vi "Compile - Rx Packet Information.vi"(8 "error in (no error)":errorcluster, 11 "Custom Device Ref in":T1 format="%.0x") -> (0 "error out":errorcluster, 1 "Rx Ref Array":T2(array[cluster]) {"VS Refs" format="%.0x"}, 2 "Rx Packet Info Array":T3[](array[typedef]) {"Endianness" items=["big-endian"=0, "little-indian"=2]}, 3 "Custom Device Ref out":T1 format="%.0x")   [LabVIEW 2019, in "UDP-Custom-Device System Explorer.lvlib"]
uses:
  UDP-Custom-Device System Explorer.lvlib
  Shared/Types/Shared - Rx.PacketInfo.ctl
  Shared/Types/Shared - Channel Data Type.ctl
  Shared/Types/Shared - Buffered.PacketInfo.ctl
  Shared/Types/Shared - Pointer Encoding.ctl
  Shared/Types/Shared - Receive Buffer Options.ctl
  Shared/Types/Shared - Transmit Buffer Options.ctl
  Shared/Types/Shared - Duplex Settings.ctl
  Shared/Types/Shared - New Data Options.ctl
  Shared/Types/Shared - Thread Management.ctl
  <vilib>/NI VeriStand/Custom Device API/Custom Device Item Ref.ctl
  Shared/UDP-Custom-Device Shared.lvlib
  <vilib>/NI VeriStand/Custom Device API/Custom Device API.lvlib
  Property Accessors/Rx Channel Accessors.lvlib
  Property Accessors/Shared Packet Accessors.lvlib
  Property Accessors/Rx Packet Accessors.lvlib
  Property Accessors/Buffered Data Packet.lvlib
  Property Accessors/Rx Channel Section Accessors.lvlib
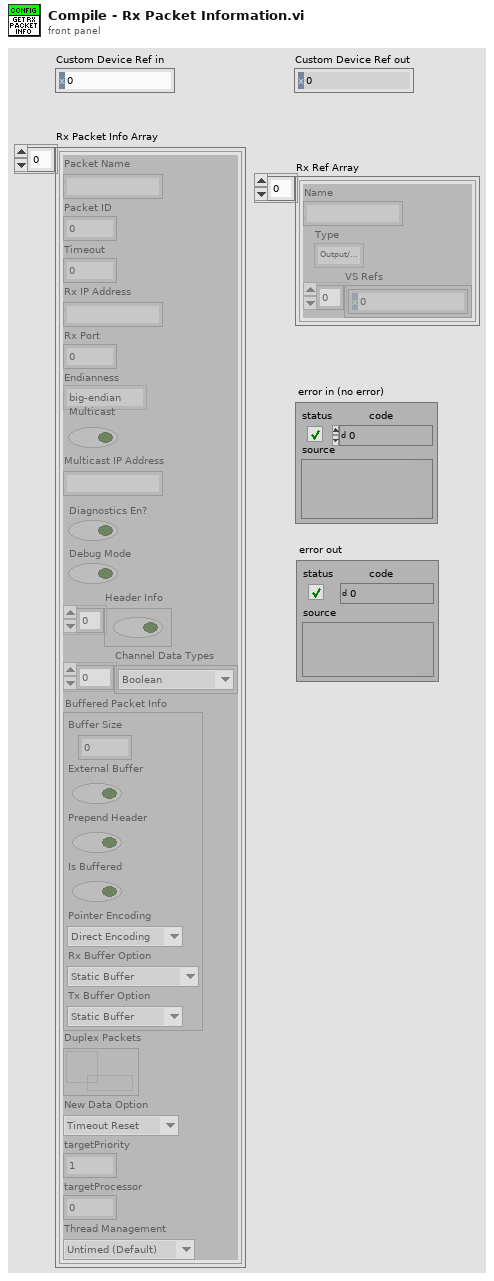
[diagram p1: front panel]
types:
  T1 = typedef "Custom Device API.lvlib/Custom Device Item Ref.ctl" = u64
  T2 = cluster{"Name":string, "Type":enum16{"Output/Write", "Input/Read", "Input/ReadWrite"}, "VS Refs":T1[]}[]
  T3 = typedef "UDP-Custom-Device Shared.lvlib/Shared - Rx.PacketInfo.ctl" = cluster{"Packet Name":string, "Packet ID":i32, "Timeout":i32, "Rx IP Address":string, "Rx Port":u16, "Endianness":u16, "Multicast":bool, "Multicast IP Address":string, "Diagnostics En?":bool, "Debug Mode":bool, "Header Info":bool[], "Channel Data Types":T4[], "Buffered Packet Info":T5, "Duplex Packets":refnum<data-value>, "New Data Option":T9, "targetPriority":i16, "targetProcessor":i8, "Thread Management":T10}
  T4 = typedef "UDP-Custom-Device Shared.lvlib/Shared - Channel Data Type.ctl" = enum16{"Boolean", "Single", "Double", "I8", "I16", "I32", "I64", "U8", "U16", "U32", "U64"}
  T5 = typedef "UDP-Custom-Device Shared.lvlib/Shared - Buffered.PacketInfo.ctl" = cluster{"Buffer Size":i32, "External Buffer":bool, "Prepend Header":bool, "Is Buffered":bool, "Pointer Encoding":T6, "Rx Buffer Option":T7, "Tx Buffer Option":T8}
  T6 = typedef "UDP-Custom-Device Shared.lvlib/Shared - Pointer Encoding.ctl" = enum16{"Direct Encoding", "Conversion Encoding"}
  T7 = typedef "UDP-Custom-Device Shared.lvlib/Shared - Receive Buffer Options.ctl" = enum16{"Static Buffer", "Circular Buffer", "Circular Buffer + Size", "Internal Cache", "Internal Cache + Size", "Ping Pong", "Ping Pong + Size"}
  T8 = typedef "UDP-Custom-Device Shared.lvlib/Shared - Transmit Buffer Options.ctl" = enum16{"Static Buffer", "FIFO Buffer", "FIFO Buffer + Port"}
  T9 = typedef "UDP-Custom-Device Shared.lvlib/Shared - New Data Options.ctl" = enum16{"Timeout Reset", "Counter"}
  T10 = typedef "UDP-Custom-Device Shared.lvlib/Shared - Thread Management.ctl" = enum16{"Untimed (Default)", "Timed (High Priority)"}
  T11 = typedef "UDP-Custom-Device System Explorer.lvlib/Packet Type.ctl" = enum16{"Transmit", "Receive", "Buffered Transmit", "Buffered Receive"}
  T12 = typedef "Custom Device API.lvlib/Custom Device Item Info.ctl" = cluster{"Name":string, "Is Channel":bool, "GUID":string, "Is Waveform":bool}
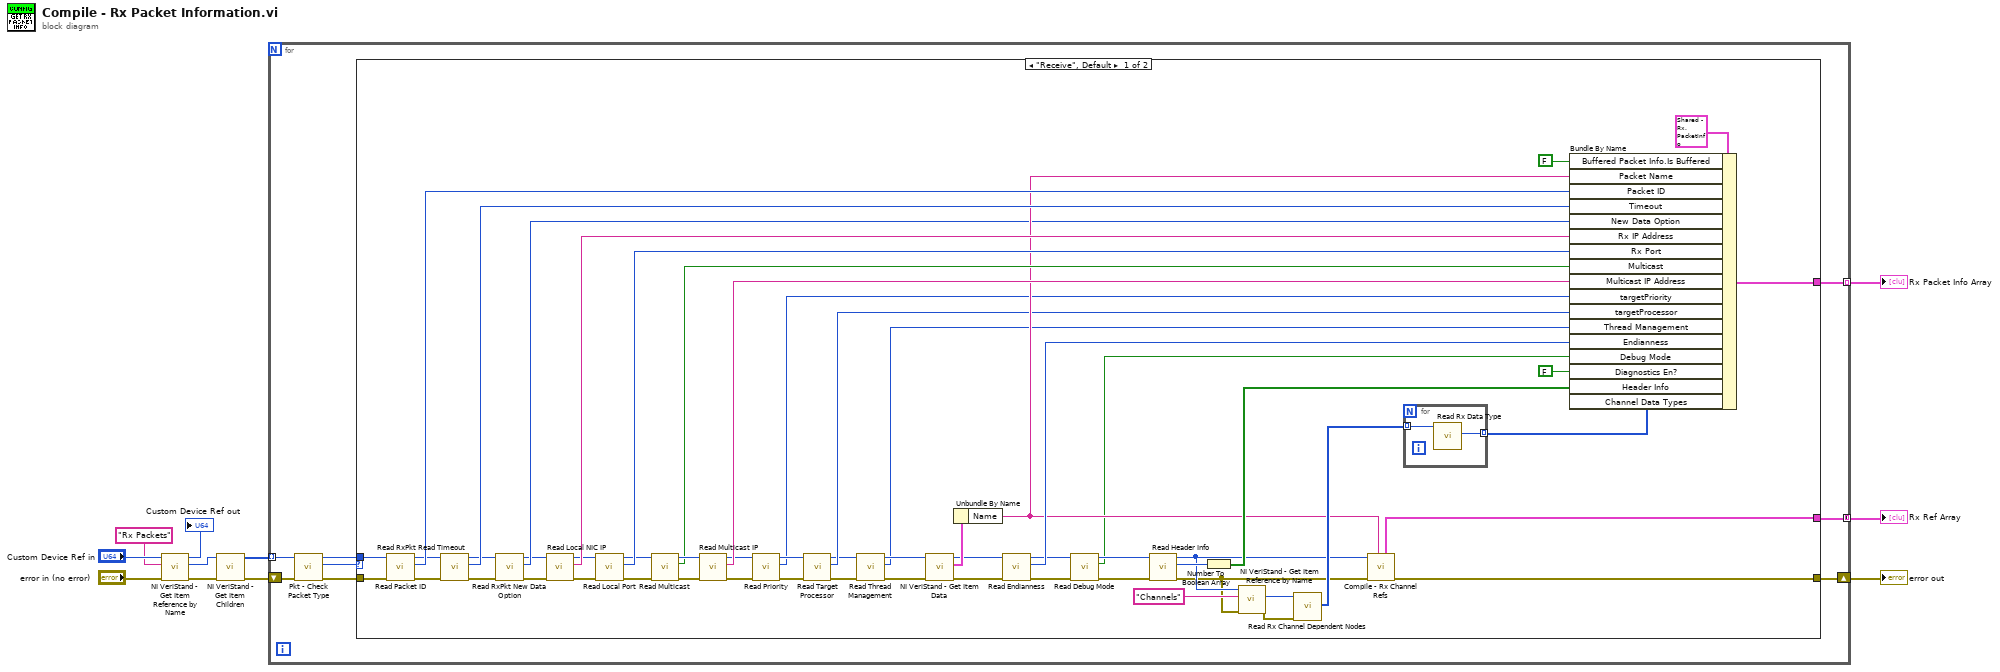
[diagram p0: block diagram]
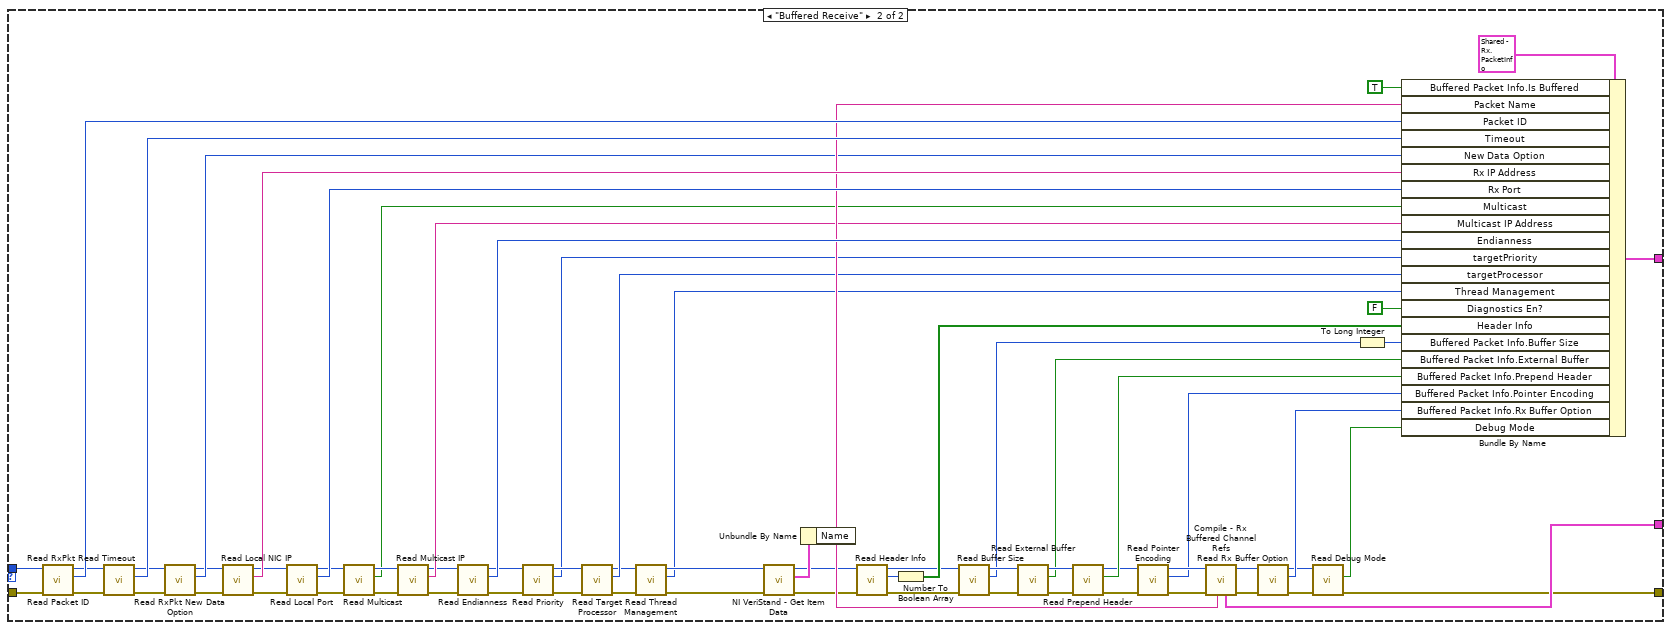
[diagram p2: hidden frame]
diagram:
  n1 = call <vilib>:"NI VeriStand - Get Item Reference by Name.vi"("error in (no error)"="error in (no error)", "Item Name"="Rx Packets", "Parent Ref in"="Custom Device Ref in") -> ("error out"=w5:errorcluster, "Item Ref"=w2:T1, "Parent Ref out"=→"Custom Device Ref out":T1)  [unwired: 5 in, 1 out]
  n2 = call <vilib>:"NI VeriStand - Get Item Children.vi"("error in (no error)"=w5, "Item Ref in"=w2) -> ("error out"=w8:errorcluster, "Child Refs"=w7:T1[])  [unwired: 6 in, 2 out]
  n3 = for {
    tunnel: w7 -> [w17] mode=indexing
    shift-right: [w18] -> w10
    shift-left: w8 -> [w15]
    tunnel: [w19] -> w9 mode=indexing
    tunnel: [w13] -> w6 mode=concatenating
    n4 = call "Pkt - Check Packet Type.vi"("error in (no error)"=w15, "Node Ptr In"=w17) -> ("error out"=w14:errorcluster, "Packet Type"=w12:T11, "Node Ptr Out"=w16:T1)  [unwired: 7 in]
    n5 = case shown="\"Receive\", Default" w12 {
      tunnel: [w75 w145] -> w19
      tunnel: [w51 w108] -> w18
      tunnel: w16 -> [w42 w106]
      tunnel: w14 -> [w41 w105]
      tunnel: [w50 w123] -> w13
      frame "Receive", Default {
        n6 = call "Read Packet ID.vi"("error in (no error)"=w41, "Node Ptr"=w42) -> ("error out"=w39:errorcluster, "Packet ID"=w65:i32, "Node Ptr out"=w40:T1)  [unwired: 7 in]
        n7 = call "Read RxPkt Read Timeout.vi"("error in (no error)"=w39, "Node Ptr"=w40) -> ("error out"=w37:errorcluster, "Read Timeout"=w66:i32, "Node Ptr out"=w38:T1)  [unwired: 7 in]
        n8 = call "Read RxPkt New Data Option.vi"("error in (no error)"=w37, "Node Ptr"=w38) -> ("error out"=w35:errorcluster, "New Data Option"=w48:T9, "Node Ptr out"=w36:T1)  [unwired: 7 in]
        n9 = call "Read Local NIC IP.vi"("error in (no error)"=w35, "Node Ptr"=w36) -> ("error out"=w33:errorcluster, "IP Address of Local NIC"=w68:string, "Node Ptr out"=w34:T1)  [unwired: 7 in]
        n10 = call "Read Local Port.vi"("error in (no error)"=w33, "Node Ptr"=w34) -> ("error out"=w31:errorcluster, "Port"=w67:u16, "Node Ptr out"=w32:T1)  [unwired: 7 in]
        n11 = call "Read Multicast.vi"("error in (no error)"=w31, "Node Ptr"=w32) -> ("error out"=w56:errorcluster, "Multicast"=w55:bool, "Node Ptr out"=w57:T1)  [unwired: 7 in]
        n12 = call "Read Multicast IP.vi"("error in (no error)"=w56, "Node Ptr"=w57) -> ("error out"=w28:errorcluster, "Multicast IP Address"=w54:string, "Node Ptr out"=w27:T1)  [unwired: 7 in]
        n13 = call "Read Priority.vi"("error in (no error)"=w28, "Node Ptr"=w27) -> ("error out"=w29:errorcluster, "targetPriority"=w26:i16, "Node Ptr out"=w30:T1)  [unwired: 7 in]
        n14 = call "Read Target Processor.vi"("error in (no error)"=w29, "Node Ptr"=w30) -> ("error out"=w22:errorcluster, "targetProcessor"=w25:i8, "Node Ptr out"=w24:T1)  [unwired: 7 in]
        n15 = call "Read Thread Management.vi"("error in (no error)"=w22, "Node Ptr"=w24) -> ("error out"=w21:errorcluster, "Thread Management"=w20:T10, "Node Ptr out"=w23:T1)  [unwired: 7 in]
        n16 = call <vilib>:"NI VeriStand - Get Item Data.vi"("error in (no error)"=w21, "Item Ref in"=w23) -> ("error out"=w61:errorcluster, "Item Info"=w64:T12, "Item Ref out"=w62:T1)  [unwired: 6 in, 1 out]
        n17 = Unbundle By Name(w64) -> ("Name"=w49:string)
        n18 = call "Read Endianness.vi"("error in (no error)"=w61, "Node Ptr"=w62) -> ("error out"=w45:errorcluster, "Endianness"=w60:u16, "Node Ptr out"=w47:T1)  [unwired: 7 in]
        n19 = call "Read Debug Mode.vi"("error in (no error)"=w45, "Node Ptr"=w47) -> ("error out"=w44:errorcluster, "Debug Mode"=w43:bool, "Node Ptr out"=w46:T1)  [unwired: 7 in]
        n20 = call "Read Header Info.vi"("error in (no error)"=w44, "Node Ptr"=w46) -> ("error out"=w52:errorcluster, "Header Info"=w59:u32, "Node Ptr out"=w53:T1)  [unwired: 7 in]
        n21 = Number To Boolean Array(number=w59) -> (Boolean array=w74:bool[])
        n22 = call <vilib>:"NI VeriStand - Get Item Reference by Name.vi"("error in (no error)"=w52, "Item Name"="Channels" ("Section Name"), "Parent Ref in"=w53) -> ("error out"=w71:errorcluster, "Item Ref"=w72:T1)  [unwired: 5 in, 2 out]
        n23 = call "Read Rx Channel Dependent Nodes.vi"("error in (no error)"=w71, "Node Ptr"=w72) -> ("Dependent Node Refs"=w70:T1[])  [unwired: 7 in, 2 out]
        n24 = call "Compile - Rx Channel Refs.vi"("Packet Name"=w49, "error in (no error)"=w52, "Item Ref in"=w53) -> ("error out"=w51:errorcluster, "Rx Ref Array"=w50:T2)  [unwired: 6 in, 1 out]
        n25 = for {
          tunnel: w70 -> [w78] mode=indexing
          tunnel: [w77] -> w69 mode=indexing
          n26 = call "Read Rx Data Type.vi"("Node Ptr"=w78) -> ("Data Type"=w77:T4)  [unwired: 8 in, 2 out]
        }
        n27 = Bundle By Name(cluster=T3 {"Packet Name"="", "Packet ID"=0, "Timeout"=0, "Rx IP Address"="", "Rx Port"=0, "Endianness"=0, "Multicast"=FALSE, "Multicast IP Address"="", "Diagnostics En?"=FALSE, "Debug Mode"=FALSE, "Header Info"=[], "Channel Data Types"=[], "Buffered Packet Info"={"Buffer Size"=0, "External Buffer"=FALSE, "Prepend Header"=FALSE, "Is Buffered"=FALSE, "Pointer Encoding"=enum."Direct Encoding", "Rx Buffer Option"=enum."Static Buffer", "Tx Buffer Option"=enum."Static Buffer"}, "Duplex Packets"=refnum, "New Data Option"=enum."Timeout Reset", "targetPriority"=1, "targetProcessor"=0, "Thread Management"=enum."Untimed (Default)"} ("Packet Info"), "Buffered Packet Info.Is Buffered"=FALSE, "Packet Name"=w49, "Packet ID"=w65, "Timeout"=w66, "New Data Option"=w48, "Rx IP Address"=w68, "Rx Port"=w67, "Multicast"=w55, "Multicast IP Address"=w54, "targetPriority"=w26, "targetProcessor"=w25, "Thread Management"=w20, "Endianness"=w60, "Debug Mode"=w43, "Diagnostics En?"=FALSE, "Header Info"=w74, "Channel Data Types"=w69) -> (w75:T3)
      }
      frame "Buffered Receive" {
        n28 = call "Read Packet ID.vi"("error in (no error)"=w105, "Node Ptr"=w106) -> ("error out"=w96:errorcluster, "Packet ID"=w141:i32, "Node Ptr out"=w97:T1)  [unwired: 7 in]
        n29 = call "Read RxPkt Read Timeout.vi"("error in (no error)"=w96, "Node Ptr"=w97) -> ("error out"=w94:errorcluster, "Read Timeout"=w142:i32, "Node Ptr out"=w95:T1)  [unwired: 7 in]
        n30 = call "Read RxPkt New Data Option.vi"("error in (no error)"=w94, "Node Ptr"=w95) -> ("error out"=w92:errorcluster, "New Data Option"=w114:T9, "Node Ptr out"=w93:T1)  [unwired: 7 in]
        n31 = call "Read Local NIC IP.vi"("error in (no error)"=w92, "Node Ptr"=w93) -> ("error out"=w90:errorcluster, "IP Address of Local NIC"=w144:string, "Node Ptr out"=w91:T1)  [unwired: 7 in]
        n32 = call "Read Local Port.vi"("error in (no error)"=w90, "Node Ptr"=w91) -> ("error out"=w103:errorcluster, "Port"=w143:u16, "Node Ptr out"=w104:T1)  [unwired: 7 in]
        n33 = call "Read Multicast.vi"("error in (no error)"=w103, "Node Ptr"=w104) -> ("error out"=w102:errorcluster, "Multicast"=w121:bool, "Node Ptr out"=w122:T1)  [unwired: 7 in]
        n34 = call "Read Multicast IP.vi"("error in (no error)"=w102, "Node Ptr"=w122) -> ("error out"=w98:errorcluster, "Multicast IP Address"=w120:string, "Node Ptr out"=w99:T1)  [unwired: 7 in]
        n35 = call "Read Endianness.vi"("error in (no error)"=w98, "Node Ptr"=w99) -> ("error out"=w86:errorcluster, "Endianness"=w138:u16, "Node Ptr out"=w87:T1)  [unwired: 7 in]
        n36 = call "Read Priority.vi"("error in (no error)"=w86, "Node Ptr"=w87) -> ("error out"=w89:errorcluster, "targetPriority"=w85:i16, "Node Ptr out"=w88:T1)  [unwired: 7 in]
        n37 = call "Read Target Processor.vi"("error in (no error)"=w89, "Node Ptr"=w88) -> ("error out"=w83:errorcluster, "targetProcessor"=w84:i8, "Node Ptr out"=w82:T1)  [unwired: 7 in]
        n38 = call "Read Thread Management.vi"("error in (no error)"=w83, "Node Ptr"=w82) -> ("error out"=w80:errorcluster, "Thread Management"=w79:T10, "Node Ptr out"=w81:T1)  [unwired: 7 in]
        n39 = call <vilib>:"NI VeriStand - Get Item Data.vi"("error in (no error)"=w80, "Item Ref in"=w81) -> ("error out"=w100:errorcluster, "Item Info"=w140:T12, "Item Ref out"=w101:T1)  [unwired: 6 in, 1 out]
        n40 = Unbundle By Name(w140) -> ("Name"=w124:string)
        n41 = call "Read Header Info.vi"("error in (no error)"=w100, "Node Ptr"=w101) -> ("error out"=w126:errorcluster, "Header Info"=w137:u32, "Node Ptr out"=w127:T1)  [unwired: 7 in]
        n42 = Number To Boolean Array(number=w137) -> (Boolean array=w135:bool[])
        n43 = call "Read Buffer Size.vi"("error in (no error)"=w126, "Node Ptr"=w127) -> ("error out"=w134:errorcluster, "Buffer Size"=w131:u32, "Node Ptr out"=w132:T1)  [unwired: 7 in]
        n44 = call "Read External Buffer.vi"("error in (no error)"=w134, "Node Ptr"=w132) -> ("error out"=w133:errorcluster, "External Buffer"=w125:bool, "Node Ptr out"=w130:T1)  [unwired: 7 in]
        n45 = call "Read Prepend Header.vi"("error in (no error)"=w133, "Node Ptr"=w130) -> ("error out"=w117:errorcluster, "Prepend Header"=w129:bool, "Node Ptr out"=w119:T1)  [unwired: 7 in]
        n46 = call "Read Pointer Encoding.vi"("error in (no error)"=w117, "Node Ptr"=w119) -> ("error out"=w116:errorcluster, "Pointer Encoding"=w115:T6, "Node Ptr out"=w118:T1)  [unwired: 7 in]
        n47 = call "Compile - Rx Buffered Channel Refs.vi"("Packet Name"=w124, "error in (no error)"=w116, "Item Ref in"=w118) -> ("error out"=w112:errorcluster, "Item Ref out"=w113:T1, "Rx Ref Array"=w123:T2)  [unwired: 6 in]
        n48 = call "Read Rx Buffer Option.vi"("error in (no error)"=w112, "Node Ptr"=w113) -> ("error out"=w109:errorcluster, "Buffer Option"=w111:T7, "Node Ptr out"=w110:T1)  [unwired: 7 in]
        n49 = call "Read Debug Mode.vi"("error in (no error)"=w109, "Node Ptr"=w110) -> ("error out"=w108:errorcluster, "Debug Mode"=w107:bool)  [unwired: 7 in, 1 out]
        n50 = To Long Integer(number=w131) -> (32bit integer=w128:i32)
        n51 = Bundle By Name(cluster=T3 {"Packet Name"="", "Packet ID"=0, "Timeout"=0, "Rx IP Address"="", "Rx Port"=0, "Endianness"=0, "Multicast"=FALSE, "Multicast IP Address"="", "Diagnostics En?"=FALSE, "Debug Mode"=FALSE, "Header Info"=[], "Channel Data Types"=[], "Buffered Packet Info"={"Buffer Size"=0, "External Buffer"=FALSE, "Prepend Header"=FALSE, "Is Buffered"=FALSE, "Pointer Encoding"=enum."Direct Encoding", "Rx Buffer Option"=enum."Static Buffer", "Tx Buffer Option"=enum."Static Buffer"}, "Duplex Packets"=refnum, "New Data Option"=enum."Timeout Reset", "targetPriority"=1, "targetProcessor"=0, "Thread Management"=enum."Untimed (Default)"} ("Packet Info"), "Buffered Packet Info.Is Buffered"=TRUE, "Packet Name"=w124, "Packet ID"=w141, "Timeout"=w142, "New Data Option"=w114, "Rx IP Address"=w144, "Rx Port"=w143, "Multicast"=w121, "Multicast IP Address"=w120, "Endianness"=w138, "targetPriority"=w85, "targetProcessor"=w84, "Thread Management"=w79, "Diagnostics En?"=FALSE, "Header Info"=w135, "Buffered Packet Info.Buffer Size"=w128, "Buffered Packet Info.External Buffer"=w125, "Buffered Packet Info.Prepend Header"=w129, "Buffered Packet Info.Pointer Encoding"=w115, "Buffered Packet Info.Rx Buffer Option"=w111, "Debug Mode"=w107) -> (w145:T3)
      }
    }
  }
  "Rx Packet Info Array" <- w9
  "error out" <- w10
  "Rx Ref Array" <- w6
